vi "Create Script.vi"(7 "Auto Run (F: Disable)":bool, 8 "error in (no error)":errorcluster, 9 "Source Code":string="smua.reset()\nsmua.source.func = smua.OUTPUT_DCAMPS\nsmua.source.rangei = 10e-3\nsmua.source.leveli = 10e-3\nsmua.source.limitv = 10 \nsmua.sense = smua.SENSE_REMOTE smua.measure.autorangev = smua.AUTORANGE_ON \nsmua.source.output = smua.OUTPUT_ON\nprint(smua.measure.r())\nsmua.source.output = smua.OUTPUT_OFF", 10 "Script Variable":string, 11 "VISA resource name":refnum<visa-resource-name>) -> (0 "error out":errorcluster, 3 "VISA resource name out":refnum<visa-resource-name>)   [LabVIEW 2019, in "Keithley 2600 Series.lvlib"]
doc: "Creates a script.\n\n<b>Note:</b>\nWhen you created and run a script that contains the command of \"print()\", you need to call the <b>Print Variable </b>VI and set the variable name to \"Nil\" to read the output data or message."
uses:
  <instrlib>/Keithley 2600 Series/Keithley 2600 Series.lvlib
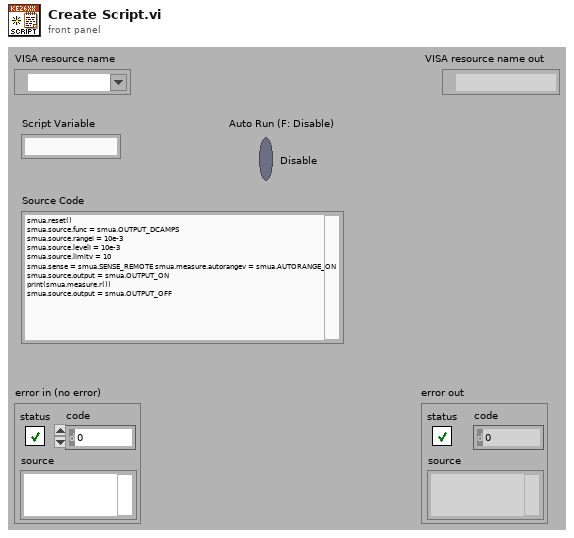
[diagram p1: front panel]
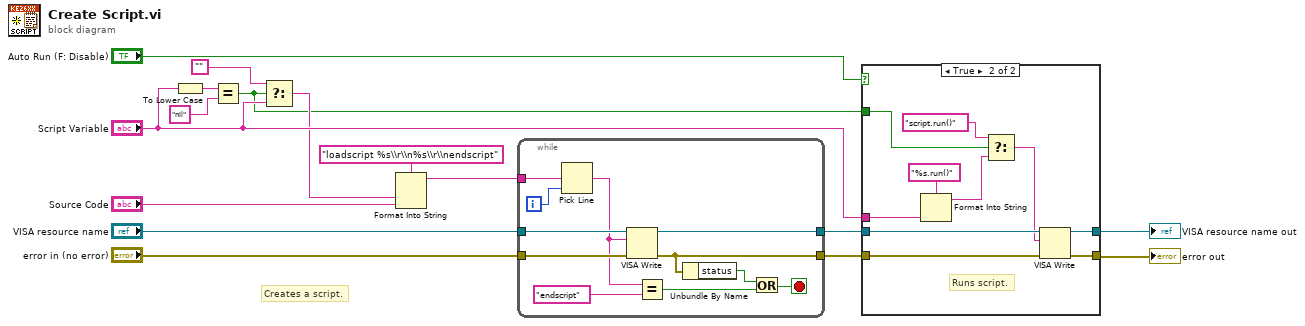
[diagram p0: block diagram]
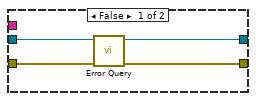
[diagram p2: hidden frame]
diagram:
  # "Creates a script."
  n1 = To Lower Case(string="Script Variable") -> (all lower case string=w8:string)
  n2 = Equal?(x=w8, y="nil") -> (x = y?=w3:bool)
  n3 = Select(t="", s=w3, f="Script Variable") -> (s? t:f=w4:string)
  n4 = Format Into String(format string="loadscript %s\\r\\n%s\\r\\nendscript", w4, "Source Code") -> (resulting string=w12:string)  [unwired: 2 in, 1 out]
  n5 = while {
    tunnel: "VISA resource name" -> [w27]
    tunnel: "error in (no error)" -> [w26]
    tunnel: [w25] -> w10
    tunnel: [w22] -> w9
    tunnel: w12 -> [w24]
    i -> [w23]
    stop <- w20 stop-if-true
    n6 = Pick Line(multi-line string=w24, line index=w23) -> (output string=w19:string)  [unwired: 1 in]
    n7 = VISA Write(VISA resource name=w27, write buffer=w19, error in (no error)=w26) -> (VISA resource name out=w25:refnum<visa-resource-name>, error out=w22:errorcluster)  [unwired: 1 out]
    n8 = Equal?(x=w19, y="endscript") -> (x = y?=w17:bool)
    n9 = Unbundle By Name(w22) -> ("status"=w21:bool)
    n10 = Or(x=w21, y=w17) -> (x .or. y?=w20:bool)
  }
  n11 = case shown="True" "Auto Run (F: Disable)" {
    tunnel: w10 -> [w31 w41]
    tunnel: w9 -> [w29 w40]
    tunnel: [w30 w39] -> w2
    tunnel: [w28 w38] -> w1
    tunnel: "Script Variable" -> [_ w36]
    tunnel: w3 -> [_ w35]
    frame False {
      n12 = call <instrlib>:"Error Query.vi"("error in (no error)"=w29, "VISA resource name"=w31) -> ("error out"=w28:errorcluster, "VISA resource name out"=w30:refnum<visa-resource-name>)  [unwired: 6 in, 2 out]
    }
    frame True {
      # "Runs script."
      n13 = Format Into String(format string="%s.run()", w36) -> (resulting string=w33:string)  [unwired: 2 in, 1 out]
      n14 = Select(t="script.run()", s=w35, f=w33) -> (s? t:f=w32:string)
      n15 = VISA Write(VISA resource name=w41, write buffer=w32, error in (no error)=w40) -> (VISA resource name out=w39:refnum<visa-resource-name>, error out=w38:errorcluster)  [unwired: 1 out]
    }
  }
  "VISA resource name out" <- w2
  "error out" <- w1
